vi "Self Test.vi"(8 "error in":errorcluster, 11 "6512 in":refnum<class "6512.lvclass">) -> (0 "error out":errorcluster, 3 "6512 out":refnum<class "6512.lvclass">)   [LabVIEW 2019, in "6512.lvlib" / "6512.lvclass"]
uses:
  Library/6512.lvclass
  Library/6512.lvclass/6512.ctl
  Accessors/Read Local Resource.vi
  builds/Instruments/DIG_IO.lvlibp/Library/DIG_IO.lvclass
  <resource>/objmgr/daqmx.rc
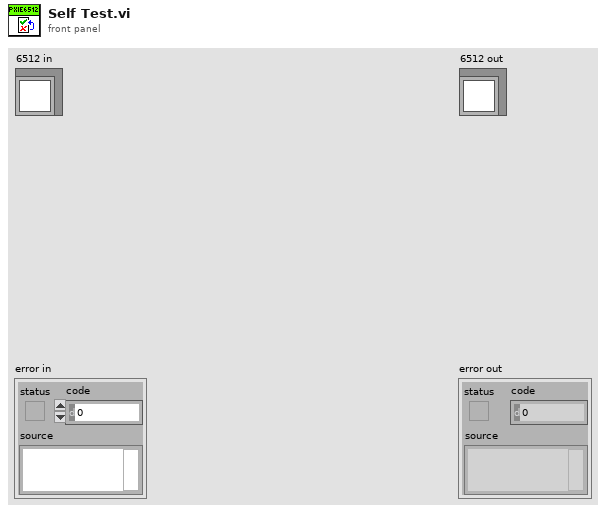
[diagram p1: front panel]
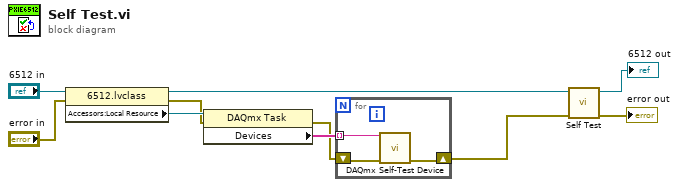
[diagram p0: block diagram]
diagram:
  n1 = property class="6512.lvclass"(reference="6512 in", error in="error in") -> (reference out=w3:refnum<class "6512.lvclass">, error out=w7:errorcluster, "Accessors:Local Resource"=w8:refnum<k21>)
  n2 = property class="DAQmx Task"(reference=w8, error in=w7) -> (error out=w5:errorcluster, "Devices"=w6:tag[])  [unwired: 1 out]
  n3 = for {
    tunnel: w6 -> [w13] mode=indexing
    shift-right: [w12] -> w4
    shift-left: w5 -> [w11]
    n4 = call <vilib>:"DAQmx Self-Test Device.vi"("device in"=w13, "error in"=w11) -> ("error out"=w12:errorcluster)  [unwired: 13 in]
  }
  n5 = call-parent "Self Test.vi"("error in"=w4, "Instruments in"=w3) -> ("error out"=→"error out":errorcluster, "Instruments out"=→"6512 out":refnum<class "6512.lvclass">)  [unwired: 8 in]
